vi "NextSlide.vi"(1 "ScanCode":i16) -> (0 "command":string)   [LabVIEW 2012]
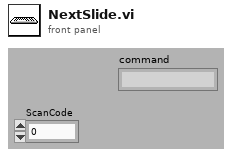
[diagram p1: front panel]
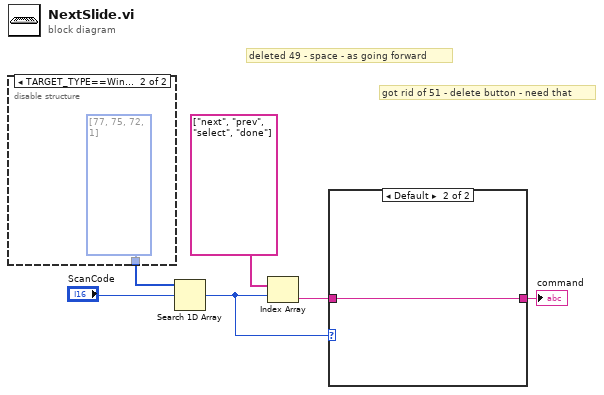
[diagram p0: block diagram]
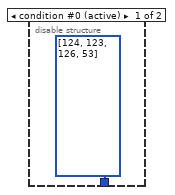
[diagram p2: hidden frame]
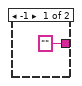
[diagram p3: hidden frame]
diagram:
  # "got rid of 51 - delete button - need that"
  # "deleted 49 - space - as going forward"
  n1 = disable-structure shown="TARGET_TYPE==Windows" {
    disable-tunnel: [i32[] [124, 123, 126, 53] i32[] [77, 75, 72, 1]] -> w6
    frame condition #0 (active) {
    }
    frame condition #1 {
    }
  }
  n2 = Search 1D Array(1D array=w6, element="ScanCode") -> (index of element=w2:i32)  [unwired: 1 in]
  n3 = Index Array(array=string[] ["next", "prev", "select", "done"], index=w2) -> (element=w3:string)
  n4 = case shown="Default" w2 {
    tunnel: w3 -> [_ w10]
    tunnel: ["" ("element") w10] -> w1
    frame -1 {
    }
    frame Default {
    }
  }
  "command" <- w1
